vi "Test Verbose Report.vi"() -> ()   [LabVIEW 2013]
uses:
  classes/Test Suite/Test Suite.lvclass
panel:
  out "error out":errorcluster
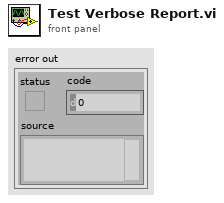
[diagram p1: front panel]
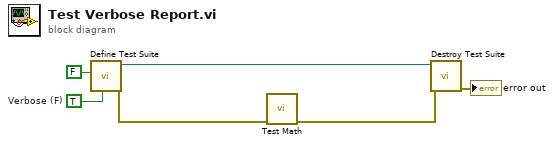
[diagram p0: block diagram]
diagram:
  w6 = TRUE  # Verbose (F)
  n1 = call "Define Test Suite.vi"("Verbose (F)"=w6, "Interactive"=FALSE) -> ("error out"=w4:errorcluster, "Test Suite"=w5:refnum<class "Test Suite.lvclass">)  [unwired: 8 in]
  n2 = call "Test Math.vi"("error in (no error)"=w4) -> ("error out"=w3:errorcluster)  [unwired: 10 in]
  n3 = call-dynamic "Destroy Test Suite.vi"("error in (no error)"=w3, "Test Suite in"=w5) -> ("error out"=→"error out":errorcluster)  [unwired: 9 in]
